vi "FindStartEndPointsHalfTrajectory.vi"() -> ()   [LabVIEW 2017]
uses:
  <vilib>/Analysis/_algsub.llb/Real Vector Norm.vi
  <vilib>/Analysis/NI_AALPro.lvlib
panel:
  out "Start Point Half Trajectory":dbl[](array[numeric])
  out "End Point Half Trajectory":dbl[](array[numeric])
  in  "threshold":dbl format="%#_13g"
  out "Nearest Collision Point":dbl[](array[numeric])
  out "Furthest Collision Point":dbl[](array[numeric])
  in  "Collision Points":dbl[][](array[numeric])
  in  "Goal":dbl[](array[numeric])
  in  "Initial State":dbl[](array[numeric])
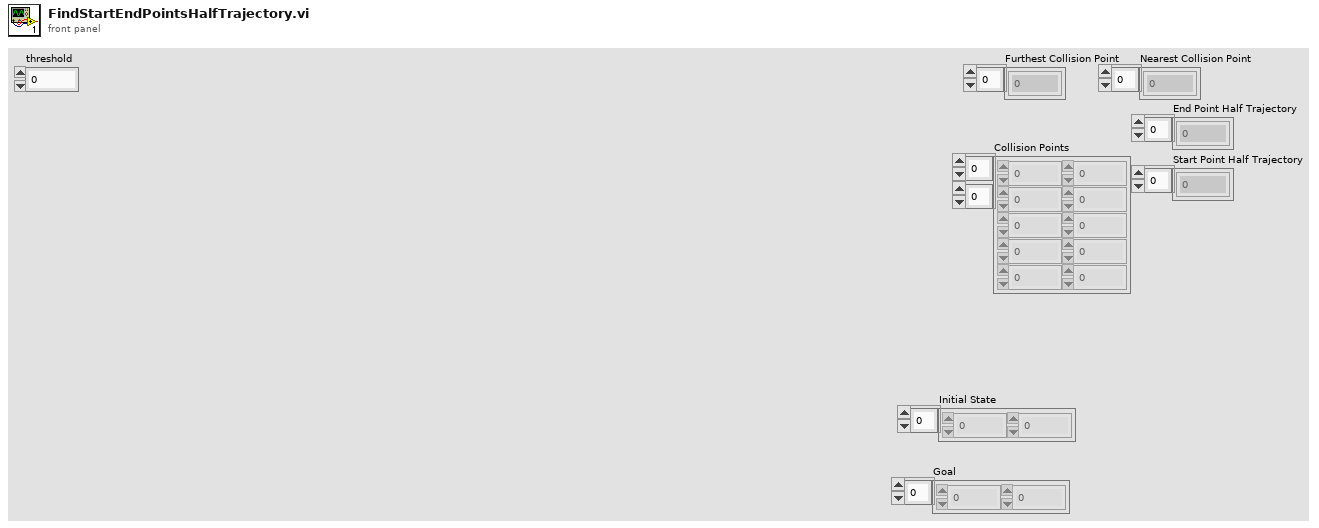
[diagram p1: front panel]
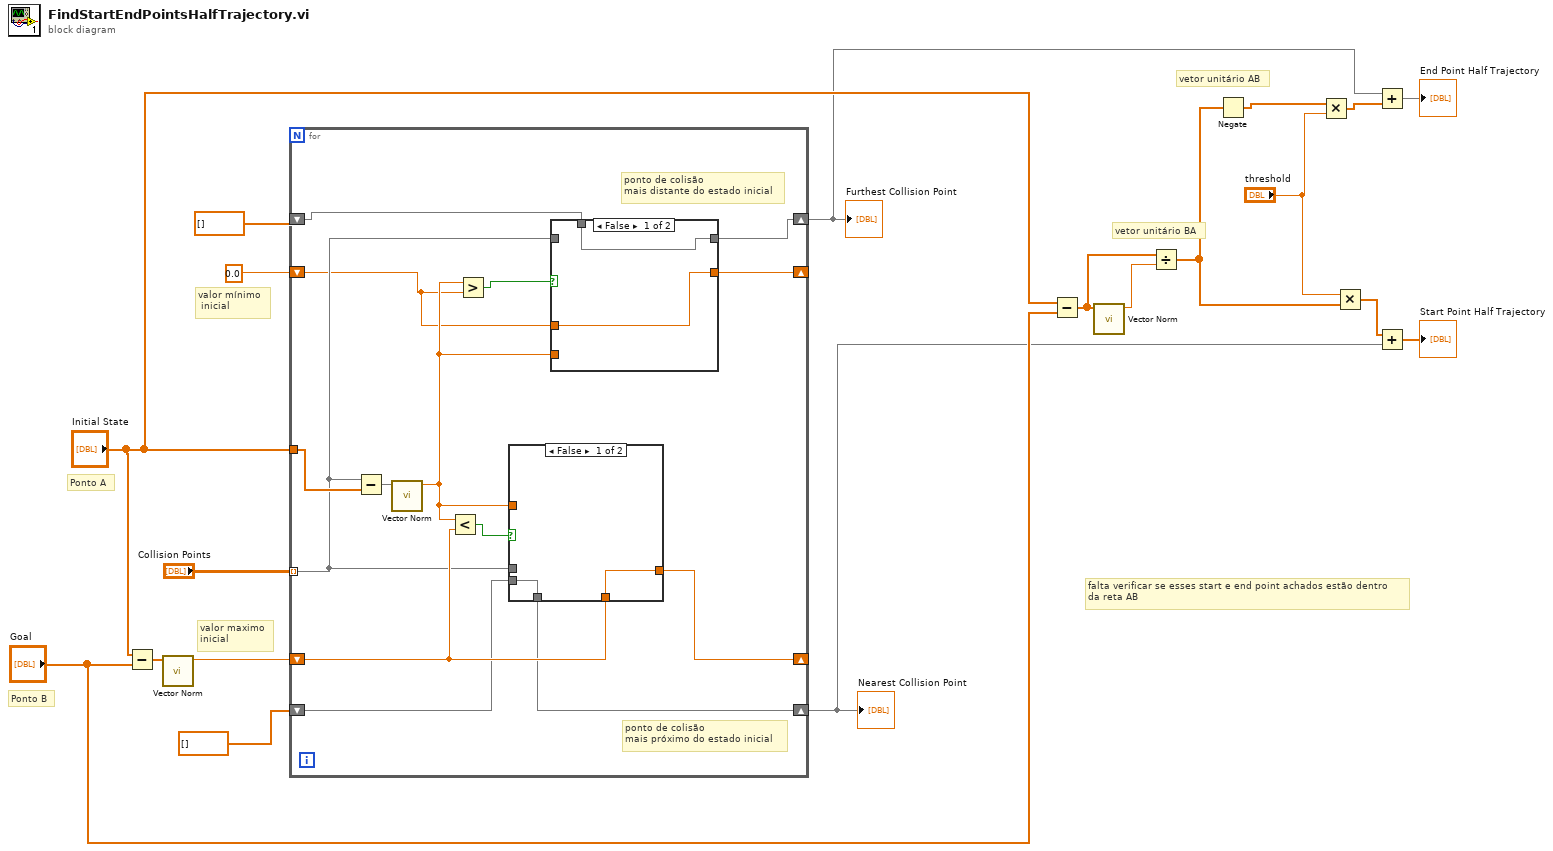
[diagram p0: block diagram]
diagram:
  # "falta verificar se esses start e end point achados estão dentro \nda reta AB"
  # "vetor unitário AB"
  # "vetor unitário BA"
  # "valor mínimo\n inicial"
  # "valor maximo\ninicial"
  # "Ponto B"
  # "Ponto A"
  n1 = Subtract(x="Initial State", y="Goal") -> (x-y=w18:dbl[])
  n2 = call-poly <vilib>:"Vector Norm.vi"("Input Vector"=w18) -> ("norm"=w17:dbl)  [unwired: 9 in, 1 out]
  n3 = for {
    tunnel: "Collision Points" -> [w23] mode=indexing
    tunnel: "Initial State" -> [w33]
    shift-right: [w24] -> _
    shift-left: 0.0 -> [w21]
    shift-right: [w29] -> _
    shift-left: w17 -> [w30]
    shift-right: [w28] -> w3
    shift-left: dbl[] [] ("Goal 2") -> [w27]
    shift-right: [w22] -> w7
    shift-left: dbl[] [] ("Goal 2") -> [w20]
    # "ponto de colisão \nmais distante do estado inicial"
    # "ponto de colisão \nmais próximo do estado inicial"
    n4 = Subtract(x=w23, y=w33) -> (x-y=w32:dbl[])
    n5 = call-poly <vilib>:"Vector Norm.vi"("Input Vector"=w32) -> ("norm"=w25:dbl)  [unwired: 9 in, 1 out]
    n6 = Less?(x=w25, y=w30) -> (x < y?=w31:bool)
    n7 = Greater?(x=w25, y=w21) -> (0:w26:bool)
    n8 = case shown="False" w31 {
      tunnel: [w39 w41] -> w29
      tunnel: w25 -> [_ w41]
      tunnel: w30 -> [w39 _]
      tunnel: w23 -> [_ w40]
      tunnel: [w38 w40] -> w28
      tunnel: w27 -> [w38 _]
      frame False {
      }
      frame True {
      }
    }
    n9 = case shown="False" w26 {
      tunnel: w25 -> [_ w37]
      tunnel: [w35 w37] -> w24
      tunnel: w23 -> [_ w36]
      tunnel: [w34 w36] -> w22
      tunnel: w21 -> [w35 _]
      tunnel: w20 -> [w34 _]
      frame False {
      }
      frame True {
      }
    }
  }
  "Furthest Collision Point" <- w7
  "Nearest Collision Point" <- w3
  n10 = Subtract(x="Initial State", y="Goal") -> (x-y=w11:dbl[])
  n11 = call-poly <vilib>:"Vector Norm.vi"("Input Vector"=w11) -> ("norm"=w10:dbl)  [unwired: 9 in, 1 out]
  n12 = Divide(x=w11, y=w10) -> (x/y=w5:dbl[])
  n13 = Negate(x=w5) -> (-x=w9:dbl[])
  n14 = Multiply(x=w9, y="threshold") -> (x*y=w8:dbl[])
  n15 = Multiply(x="threshold", y=w5) -> (x*y=w4:dbl[])
  n16 = Add(x=w7, y=w8) -> (x+y=→"End Point Half Trajectory":dbl[])
  n17 = Add(x=w4, y=w3) -> (x+y=→"Start Point Half Trajectory":dbl[])
